vi "Read SessionMailbox.vi"(8 "error in (no error)":errorcluster, 11 "Subscription in":refnum<class "Subscription.lvclass">) -> (0 "error out":errorcluster, 2 "SessionMailbox":refnum<queue>, 3 "Subscription out":refnum<class "Subscription.lvclass">)   [LabVIEW 2013, in "MQTT Server.lvlib" / "Subscription.lvclass"]
uses:
  Subscription.lvclass
  MQTT_Base/Response -- cluster.ctl
  Control Packets/ControlPacket/ControlPacket.lvclass
  Subscription.lvclass/Subscription.ctl
  MQTT_Base/MQTT_Base.lvclass
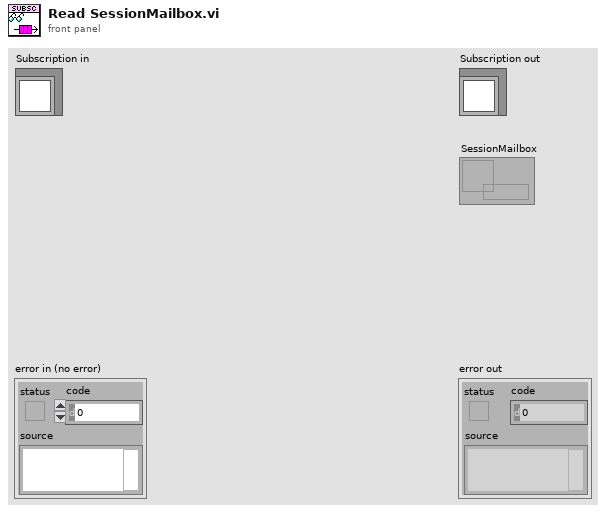
[diagram p1: front panel]
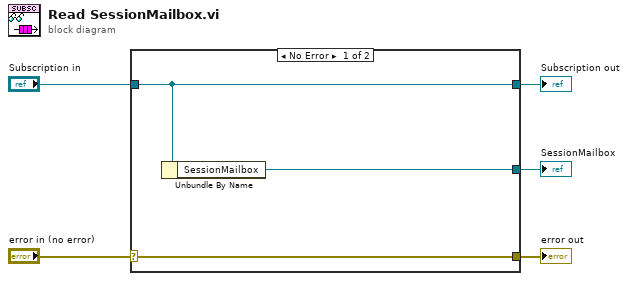
[diagram p0: block diagram]
diagram:
  n1 = case shown="No Error" "error in (no error)" {
    selector: "error in (no error)" -> [w8 w9]
    tunnel: [w8 w9] -> w4
    tunnel: [w7 w10] -> w2
    tunnel: "Subscription in" -> [w7 w10]
    tunnel: [w6 _] -> w1
    frame No Error {
      n2 = Unbundle By Name(w7) -> ("SessionMailbox"=w6:refnum<queue>)
    }
    frame Error {
    }
  }
  "error out" <- w4
  "Subscription out" <- w2
  "SessionMailbox" <- w1
